vi "Create.vi"(8 "error in (no error)":errorcluster, 11 "InterfaceLogFactory in":refnum<class "InterfaceLogFactory.lvclass">) -> (0 "error out":errorcluster, 2 "InterfaceLog":refnum<class "InterfaceLog.lvclass">, 3 "InterfaceLogFactory out":refnum<class "InterfaceLogFactory.lvclass">)   [LabVIEW 2016, in "InterfaceLogFactory.lvclass"]
uses:
  InterfaceLogFactory.lvclass
  InterfaceLog.lvclass
  common_configurationreader/ConfigurationReader.lvclass
  Typedefs/LogPath.ctl
  View/M1M3SupportEUI_View.vi
  View/M1M3SupportEUI_Views.lvlib
  Typedefs/M1M3SupportEUI_TypeDefs.lvlib
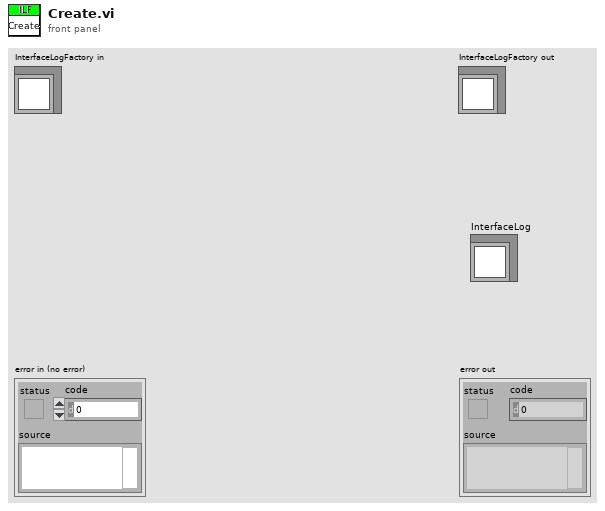
[diagram p1: front panel]
types:
  T1 = typedef "M1M3SupportEUI_TypeDefs.lvlib/LogPath.ctl" = path
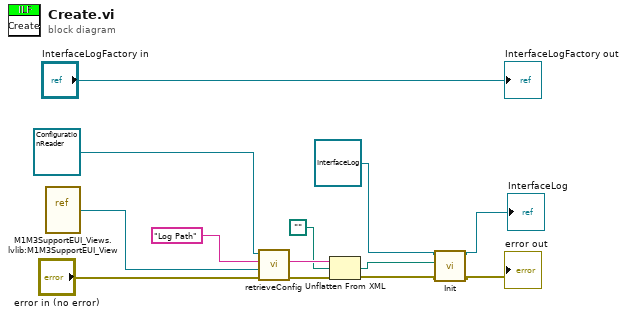
[diagram p0: block diagram]
diagram:
  n1 = vi-ref "M1M3SupportEUI_Views.lvlib:M1M3SupportEUI_View.vi"() -> (w10:refnum<vi>)
  n2 = call "retrieveConfig.vi"("error in (no error)"="error in (no error)", "callingVIRef"=w10, "configName"="Log Path", "ConfigurationReader in"=refnum<class "ConfigurationReader.lvclass"> refnum ("ConfigurationReader.lvclass")) -> ("error out"=w8:errorcluster, "xmlData"=w7:string)  [unwired: 5 in, 1 out]
  n3 = Unflatten From XML(xml string=w7, type=T1 path "" ("Log Path"), error in (no error)=w8) -> (value=w1:T1, error out=w5:errorcluster)
  n4 = call "Init.vi"("InterfaceLog in"=refnum<class "InterfaceLog.lvclass"> refnum ("InterfaceLog.lvclass"), "Log Path"=w1, "error in (no error)"=w5) -> ("InterfaceLog out"=→"InterfaceLog":refnum<class "InterfaceLog.lvclass">, "error out"=→"error out":errorcluster)  [unwired: 6 in]
  "InterfaceLogFactory out" <- "InterfaceLogFactory in"
